vi "Delete Tree Item If No Longer Needed.vi"(8 "error in":errorcluster, 10 "Item Tag":string, 11 "Tree Ref":refnum<vi>) -> (0 "error out":errorcluster)   [LabVIEW 2013, in "LVTM.lvlib"]
uses:
  LVTM.lvlib
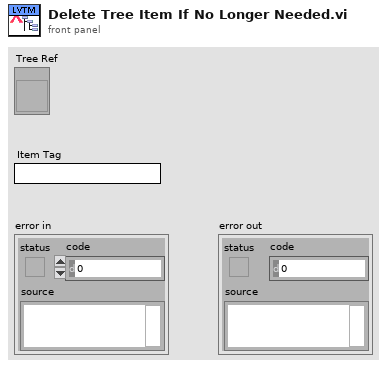
[diagram p1: front panel]
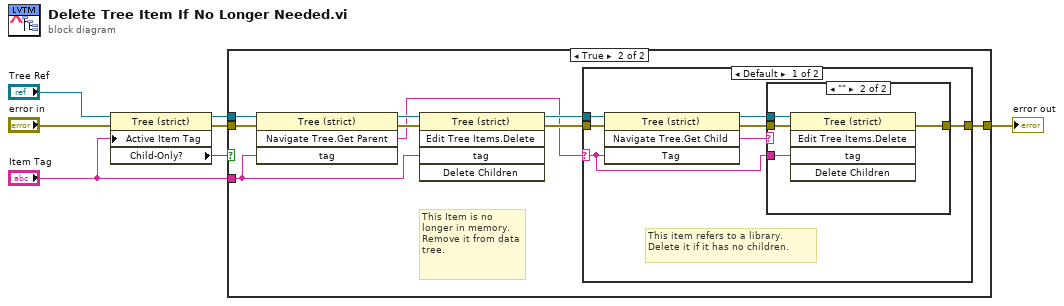
[diagram p0: block diagram]
diagram:
  n1 = property on="Property Node" class="Tree (strict)"(reference="Tree Ref", error in="error in", "Active Item Tag"="Item Tag") -> (reference out=w4:refnum<vi>, error out=w2:errorcluster, "Child-Only?"=w3:bool)
  n2 = case shown="True" w3 {
    tunnel: [w8 w10] -> w7
    tunnel: w4 -> [_ w16]
    tunnel: "Item Tag" -> [_ w17]
    tunnel: w2 -> [w8 w15]
    frame False {
      # "This item refers to a library. \nDelete it only if all items under it have left memory and have been already deleted.\nSo, do this in the other case."
    }
    frame True {
      # "This Item is no longer in memory. Remove it from data tree."
      n3 = invoke on="Invoke Node" class="Tree (strict)" method="Navigate Tree.Get Parent"(reference=w16, error in=w15, "tag"=w17) -> (reference out=w14:refnum<vi>, error out=w13:errorcluster, "Navigate Tree:Get Parent"=w9:string)  [unwired: 1 in, 1 out]
      n4 = invoke on="Invoke Node" class="Tree (strict)" method="Edit Tree Items.Delete"(reference=w14, error in=w13, "tag"=w17) -> (reference out=w11:refnum<vi>, error out=w12:errorcluster)  [unwired: 2 in, 3 out]
      n5 = case shown="Default" w9 {
        selector: w9 -> [w18 _]
        tunnel: w12 -> [w24 w30]
        tunnel: w11 -> [w23 _]
        tunnel: [w20 w30] -> w10
        frame Default {
          # "This item refers to a library. \nDelete it if it has no children."
          n6 = invoke on="Invoke Node" class="Tree (strict)" method="Navigate Tree.Get Child"(reference=w23, error in=w24, "Tag"=w18) -> (reference out=w22:refnum<vi>, error out=w21:errorcluster, "Navigate Tree:Get Child"=w19:string)  [unwired: 1 in, 1 out]
          n7 = case shown="\"\"" w19 {
            tunnel: w22 -> [_ w29]
            tunnel: w21 -> [w25 w28]
            tunnel: [w25 w27] -> w20
            tunnel: w18 -> [_ w26]
            frame Default {
            }
            frame "" {
              n8 = invoke on="Invoke Node" class="Tree (strict)" method="Edit Tree Items.Delete"(reference=w29, error in=w28, "tag"=w26) -> (error out=w27:errorcluster)  [unwired: 2 in, 4 out]
            }
          }
        }
        frame "" {
        }
      }
    }
  }
  "error out" <- w7
